vi "Get Temperature.vi"(7 "VISA resource":refnum<visa-resource-name>, 8 "error in (no error)":errorcluster, 9 "Name":string, 10 "Data":T1={"Record heater"=FALSE, "Record RAW"=FALSE, "Set point"=0.0, "Heater range"=0.0, "Approach"=enum."Instant", "Ramp rate, K/min"=1.0, "Record Channels"=[], "Settling time "=60.0, "Settling range"=0.1, "P"=0.0, "I"=0.0, "D"=0.0, "Temperature Control"=FALSE}, 11 "LakeShore T Controller in":refnum<class "LakeShore T Controller.lvclass">) -> (0 "error out":errorcluster, 1 "Channel data":dbl[](array[numeric]), 2 "Channel names":string[](array[string]), 3 "LakeShore T Controller out":refnum<class "LakeShore T Controller.lvclass">, 4 "Controled temperature":dbl, 5 "VISA resource out":refnum<visa-resource-name>)   [LabVIEW 2015, in "LakeShore T Controller.lvclass"]
uses:
  LakeShore T Controller.lvclass
  Temperarture Controller/T controller parameters.ctl
  Instruments/Neocera/Neocera Set Point Aproach.ctl
panel:
  # "Temperature Monitor"
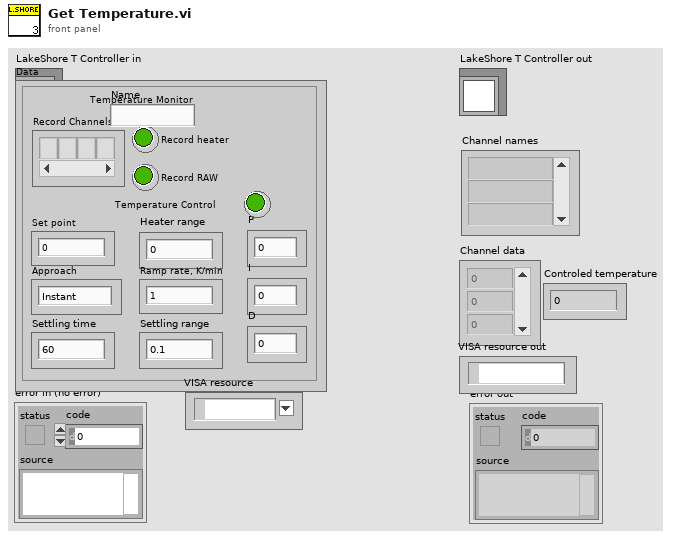
[diagram p1: front panel]
types:
  T1 = typedef "T controller parameters.ctl" = cluster{"Record heater":bool, "Record RAW":bool, "Set point":dbl, "Heater range":dbl, "Approach":T2, "Ramp rate, K/min":dbl, "Record Channels":string[], "Settling time ":dbl, "Settling range":dbl, "P":dbl, "I":dbl, "D":dbl, "Temperature Control":bool}
  T2 = typedef "Neocera Set Point Aproach.ctl" = enum16{"Instant", "Ramp"}
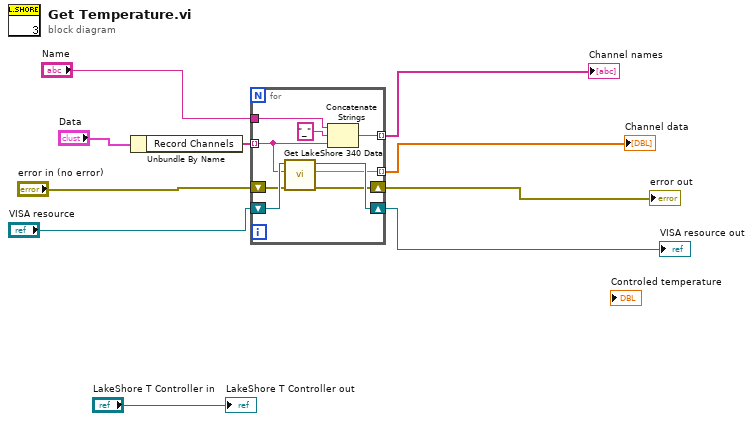
[diagram p0: block diagram]
diagram:
  n1 = Unbundle By Name("Data") -> ("Record Channels"=w10:string[])
  n2 = for {
    tunnel: [w16] -> w7 mode=indexing
    shift-right: [w19] -> w4
    shift-left: "VISA resource" -> [w18]
    shift-right: [w17] -> w3
    shift-left: "error in (no error)" -> [w15]
    tunnel: w10 -> [w12] mode=indexing
    tunnel: "Name" -> [w14]
    tunnel: [w11] -> w8 mode=indexing
    n3 = call "Get LakeShore 340 Data.vi"("error in (no error)"=w15, "Input (A or B)"=w12, "VISA Resource Name"=w18) -> ("error out"=w17:errorcluster, "Temperature"=w16:dbl, "VISA Resource Name Out"=w19:refnum<visa-resource-name>)  [unwired: 6 out]
    n4 = Concatenate Strings(w14, "_" ("string"), w12) -> (w11:string)
  }
  "error out" <- w3
  "Channel data" <- w7
  "Channel names" <- w8
  "VISA resource out" <- w4
  "LakeShore T Controller out" <- "LakeShore T Controller in"
